vi "Roots.vi"() -> ()   [LabVIEW 2024]
panel:
  out "output variable 2":cxt
  in  "input variable 3":dbl
  in  "input variable 2":dbl
  in  "input variable":dbl
  out "output variable":cxt
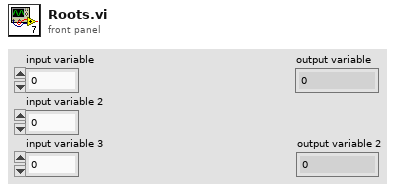
[diagram p1: front panel]
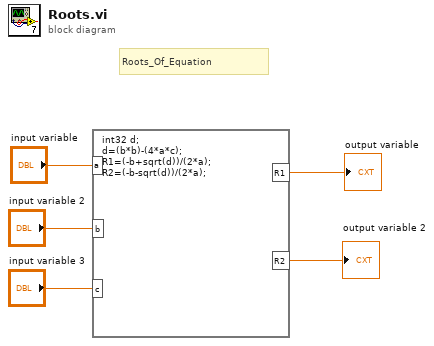
[diagram p0: block diagram]
diagram:
  # "Roots_Of_Equation"
  n1 = formula code="int32 d;\nd=(b*b)-(4*a*c);\nR1=(-b+sqrt(d))/(2*a);\nR2=(-b-sqrt(d))/(2*a);"("a"="input variable", "b"="input variable 2", "c"="input variable 3") -> ("R1"=→"output variable":dbl, "R2"=→"output variable 2":dbl)
